vi "Add FPGA.vi"(6 "FPGA Target":T2, 8 "error in (no error)":errorcluster, 10 "Bitfile Path":path, 11 "Item Ref in":T1 format="%.0x") -> (0 "error out":errorcluster, 3 "Item Ref out":T1 format="%.0x")   [LabVIEW 2019, in "SEECD System Explorer.lvlib"]
uses:
  SEECD System Explorer.lvlib
  <vilib>/NI VeriStand/Custom Device API/Custom Device Item Ref.ctl
  Type Defs/FPGA Target.ctl
  <vilib>/NI VeriStand/Custom Device API/Custom Device API.lvlib
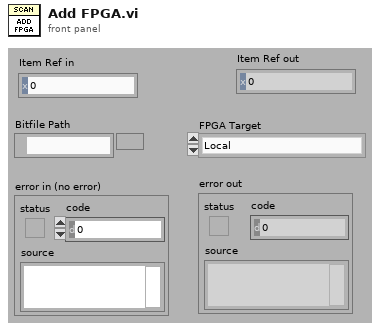
[diagram p1: front panel]
types:
  T1 = typedef "Custom Device API.lvlib/Custom Device Item Ref.ctl" = u64
  T2 = typedef "SEECD System Explorer.lvlib/FPGA Target.ctl" = enum16{"Local", "EtherCAT"}
  T3 = typedef "SEECD System Explorer.lvlib/Bitfile Signature.ctl" = cluster{"Signature (Hex) - Local FPGA":string, "Signature (SDO) - New ECAT API":u32, "Signature (XML) - Old ECAT API":u32}
  T4 = cluster{"name":string, "read":bool, "address":u32, "signed":bool, "size":u32, "datatype":string, "integersize":i32}[]
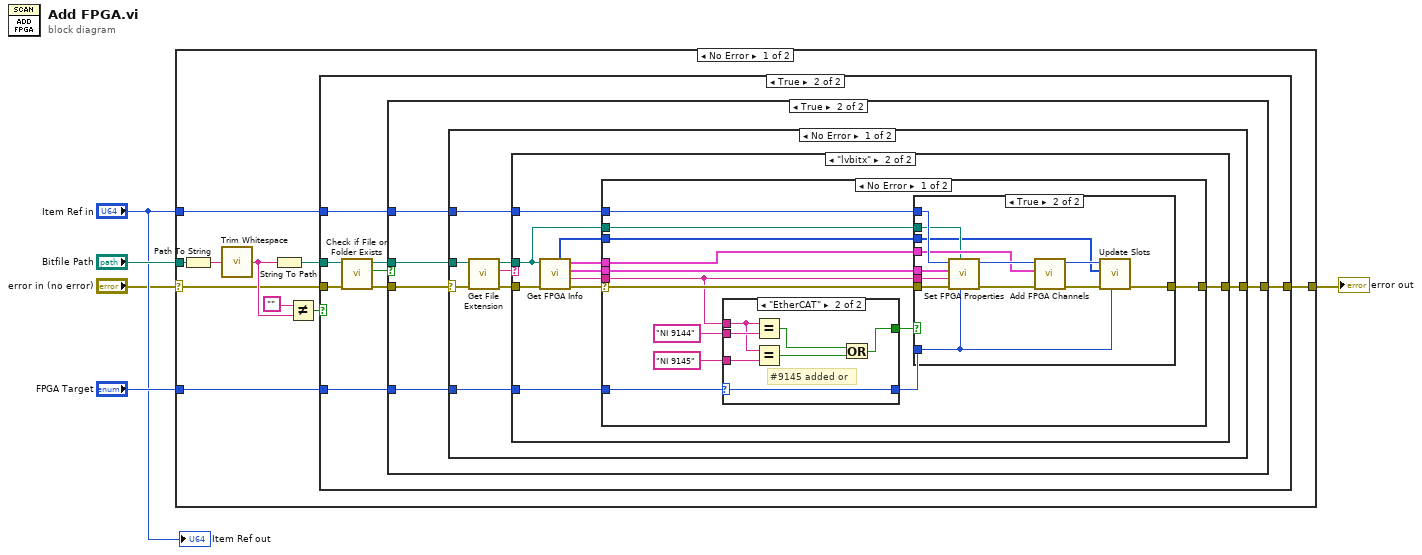
[diagram p0: block diagram]
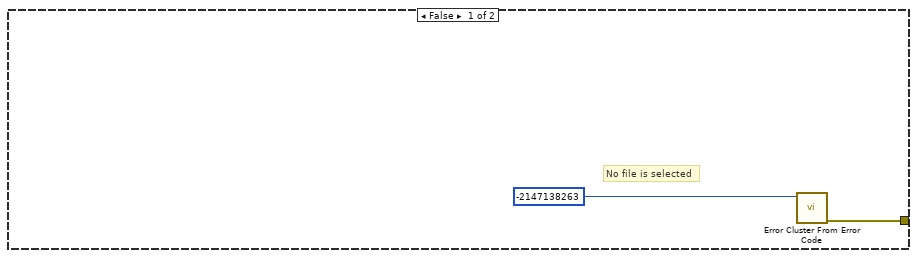
[diagram p2: hidden frame]
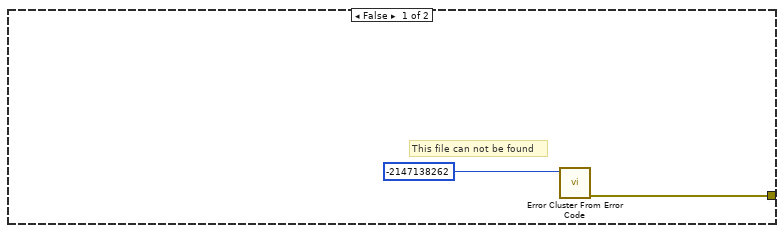
[diagram p3: hidden frame]
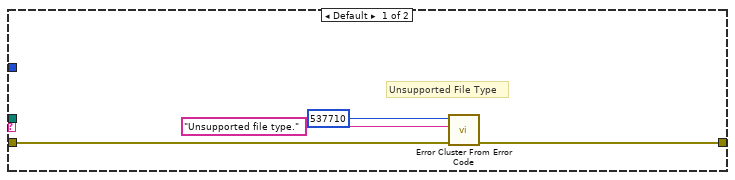
[diagram p4: hidden frame]
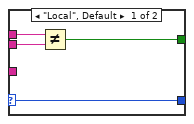
[diagram p5: hidden frame]
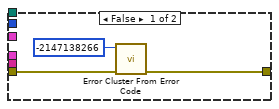
[diagram p6: hidden frame]
diagram:
  n1 = case shown="No Error" "error in (no error)" {
    selector: "error in (no error)" -> [w6 w97]
    tunnel: [w15 w97] -> w1
    tunnel: "Bitfile Path" -> [w14 _]
    tunnel: "FPGA Target" -> [w8 _]
    tunnel: "Item Ref in" -> [w7 _]
    frame No Error {
      n2 = Path To String(path=w14) -> (string=w11:string)
      n3 = call <vilib>:"Trim Whitespace.vi"("string"=w11) -> ("trimmed string"=w9:string)  [unwired: 1 in]
      n4 = String To Path(string=w9) -> (path=w13:path)
      n5 = Not Equal?(x="", y=w9) -> (x != y?=w12:bool)
      n6 = case shown="True" w12 {
        tunnel: w13 -> [_ w25]
        tunnel: [w16 w21] -> w15
        tunnel: w6 -> [_ w20]
        tunnel: w8 -> [_ w19]
        tunnel: w7 -> [_ w18]
        frame False {
          # "No file is selected"
          n7 = call <vilib>:"Error Cluster From Error Code.vi"("error code (0)"=-2147138263) -> ("error out"=w16:errorcluster)  [unwired: 8 in]
        }
        frame True {
          n8 = call <vilib>:"Check if File or Folder Exists.vi"("error in (no error)"=w20, "path"=w25) -> ("error out"=w23:errorcluster, "file or folder exists?"=w24:bool, "dup path"=w22:path)  [unwired: 7 out]
          n9 = case shown="True" w24 {
            tunnel: w23 -> [_ w31]
            tunnel: w22 -> [_ w32]
            tunnel: [w26 w30] -> w21
            tunnel: w19 -> [_ w29]
            tunnel: w18 -> [_ w28]
            frame False {
              # "This file can not be found"
              n10 = call <vilib>:"Error Cluster From Error Code.vi"("error code (0)"=-2147138262) -> ("error out"=w26:errorcluster)  [unwired: 8 in]
            }
            frame True {
              n11 = case shown="No Error" w31 {
                selector: w31 -> [w39 w96]
                tunnel: w32 -> [w40 _]
                tunnel: [w36 w96] -> w30
                tunnel: w29 -> [w34 _]
                tunnel: w28 -> [w33 _]
                frame No Error {
                  n12 = call <vilib>:"Get File Extension.vi"("error in (no error)"=w39, "file"=w40) -> ("error out"=w37:errorcluster, "lowercase file extension"=w38:string, "dup file"=w35:path)  [unwired: 7 out]
                  n13 = case shown="\"lvbitx\"" w38 {
                    tunnel: w37 -> [w44 w53]
                    tunnel: w35 -> [_ w47]
                    tunnel: [w43 w49] -> w36
                    tunnel: w34 -> [_ w48]
                    tunnel: w33 -> [_ w46]
                    frame Default {
                      # "Unsupported File Type"
                      n14 = call <vilib>:"Error Cluster From Error Code.vi"("error in (no error)"=w44, "error message (\"\")"="Unsupported file type." ("error message (\"\")"), "error code (0)"=537710) -> ("error out"=w43:errorcluster)  [unwired: 6 in]
                    }
                    frame "lvbitx" {
                      n15 = call "Get FPGA Info.vi"("error in"=w53, "Input bitfile path"=w47) -> ("error out"=w54:errorcluster, "TargetClass"=w52:string, "Signature"=w51:T3, "User defined IOVs"=w50:T4, "Scan Mode Slots"=w45:u32[])  [unwired: 5 in]
                      n16 = case shown="No Error" w54 {
                        selector: w54 -> [w65 w95]
                        tunnel: w52 -> [w61 _]
                        tunnel: w51 -> [w66 _]
                        tunnel: w50 -> [w67 _]
                        tunnel: [w64 w95] -> w49
                        tunnel: w48 -> [w60 _]
                        tunnel: w47 -> [w58 _]
                        tunnel: w46 -> [w57 _]
                        tunnel: w45 -> [w56 _]
                        frame No Error {
                          n17 = case shown="\"EtherCAT\"" w60 {
                            selector: w60 -> [w68 w77]
                            tunnel: [w71 w76] -> w63
                            tunnel: "NI 9144" ("y") -> [w70 w78]
                            tunnel: w61 -> [w69 w73]
                            tunnel: [w68 w77] -> w59
                            tunnel: "NI 9145" ("y") -> [_ w74]
                            frame "Local", Default {
                              n18 = Not Equal?(x=w69, y=w70) -> (x != y?=w71:bool)
                            }
                            frame "EtherCAT" {
                              # "#9145 added or"
                              n19 = Equal?(x=w73, y=w78) -> (x = y?=w75:bool)
                              n20 = Equal?(x=w73, y=w74) -> (x = y?=w72:bool)
                              n21 = Or(x=w75, y=w72) -> (x .or. y?=w76:bool)
                            }
                          }
                          n22 = case shown="True" w63 {
                            tunnel: w67 -> [_ w88]
                            tunnel: w66 -> [_ w94]
                            tunnel: w65 -> [w80 w92]
                            tunnel: [w79 w85] -> w64
                            tunnel: w61 -> [_ w93]
                            tunnel: w59 -> [_ w82]
                            tunnel: w58 -> [_ w87]
                            tunnel: w57 -> [_ w91]
                            tunnel: w56 -> [_ w83]
                            frame False {
                              n23 = call <vilib>:"Error Cluster From Error Code.vi"("error in (no error)"=w80, "error code (0)"=-2147138266) -> ("error out"=w79:errorcluster)  [unwired: 7 in]
                            }
                            frame True {
                              n24 = call "Set FPGA Properties.vi"("FPGA Target"=w82, "Bitfile Path"=w87, "error in (no error)"=w92, "TargetClass"=w93, "Signature"=w94, "Item Ref in"=w91) -> ("error out"=w89:errorcluster, "Item Ref out"=w90:T1)  [unwired: 4 in]
                              n25 = call "Add FPGA Channels.vi"("error in (no error)"=w89, "User defined IOVs"=w88, "Item Ref in"=w90) -> ("error out"=w86:errorcluster, "Item Ref out"=w84:T1)  [unwired: 6 in]
                              n26 = call "Update Slots.vi"("FPGA Target"=w82, "error in (no error)"=w86, "Scan Mode Slots"=w83, "Item Ref in"=w84) -> ("error out"=w85:errorcluster)  [unwired: 6 in, 1 out]
                            }
                          }
                        }
                        frame Error {
                        }
                      }
                    }
                  }
                }
                frame Error {
                }
              }
            }
          }
        }
      }
    }
    frame Error {
    }
  }
  "error out" <- w1
  "Item Ref out" <- "Item Ref in"
